vi "Minimum lvlibp Compatible Version.vi"(8 "Error in":errorcluster caption="Error in (no error)") -> (0 "Error out":errorcluster, 3 "String":string="2025.09.10.000")   [LabVIEW 2017, in "Communicable State Machine.lvlib"]
uses:
  Communicable State Machine.lvlib
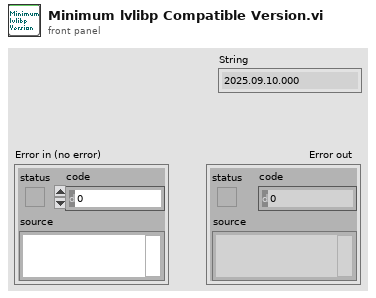
[diagram p1: front panel]
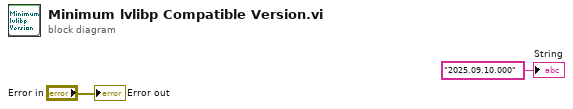
[diagram p0: block diagram]
diagram:
  "String" <- "2025.09.10.000"
  "Error out" <- "Error in"
